vi "Page_Dialog_Read.vi"(6 "ctlReferences":T1, 8 "error in (no error)":errorcluster, 11 "Class in":refnum<class "IB_MSI.lvclass">) -> (0 "error out":errorcluster, 3 "Class out":refnum<class "IB_MSI.lvclass">)   [LabVIEW 2020, in "IB_MSI.lvclass"]
uses:
  <vilib>/AppBuilder/IB_Classes/MSI/IB_MSI.lvclass
  <vilib>/AppBuilder/IB_Classes/MSI/IB_MSI.lvclass/IB_MSI.ctl
  <vilib>/AppBuilder/IB_Classes/Installer/Installer.lvclass
  <resource>/Framework/Providers/Builds/Installer/CDK_sTypeDef_Languages.ctl
  <resource>/Framework/Providers/Builds/Installer/Pages/controls/IB_UI_Page_Dialog_Info_References.ctl
  <resource>/Framework/Providers/Common/provcom_BrowseProjectFile2.ctl
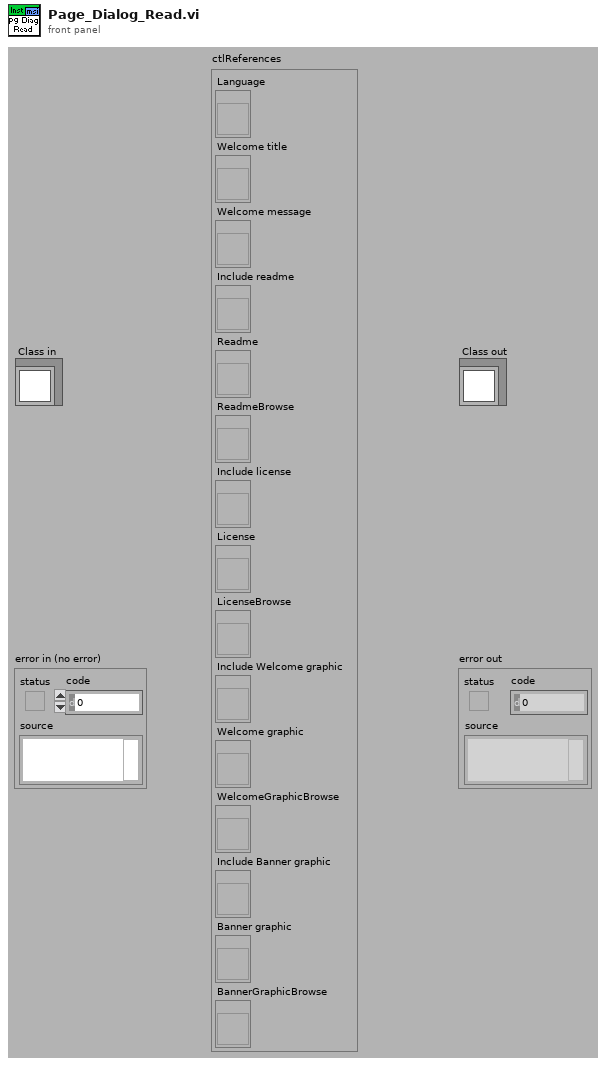
[diagram p1: front panel]
types:
  T1 = typedef "IB_UI_Page_Dialog_Info_References.ctl" = cluster{"Language":refnum<vi>, "Welcome title":refnum<vi>, "Welcome message":refnum<vi>, "Include readme":refnum<vi>, "Readme":refnum<vi>, "ReadmeBrowse":refnum<vi>, "Include license":refnum<vi>, "License":refnum<vi>, "LicenseBrowse":refnum<vi>, "Include Welcome graphic":refnum<vi>, "Welcome graphic":refnum<vi>, "WelcomeGraphicBrowse":refnum<vi>, "Include Banner graphic":refnum<vi>, "Banner graphic":refnum<vi>, "BannerGraphicBrowse":refnum<vi>}
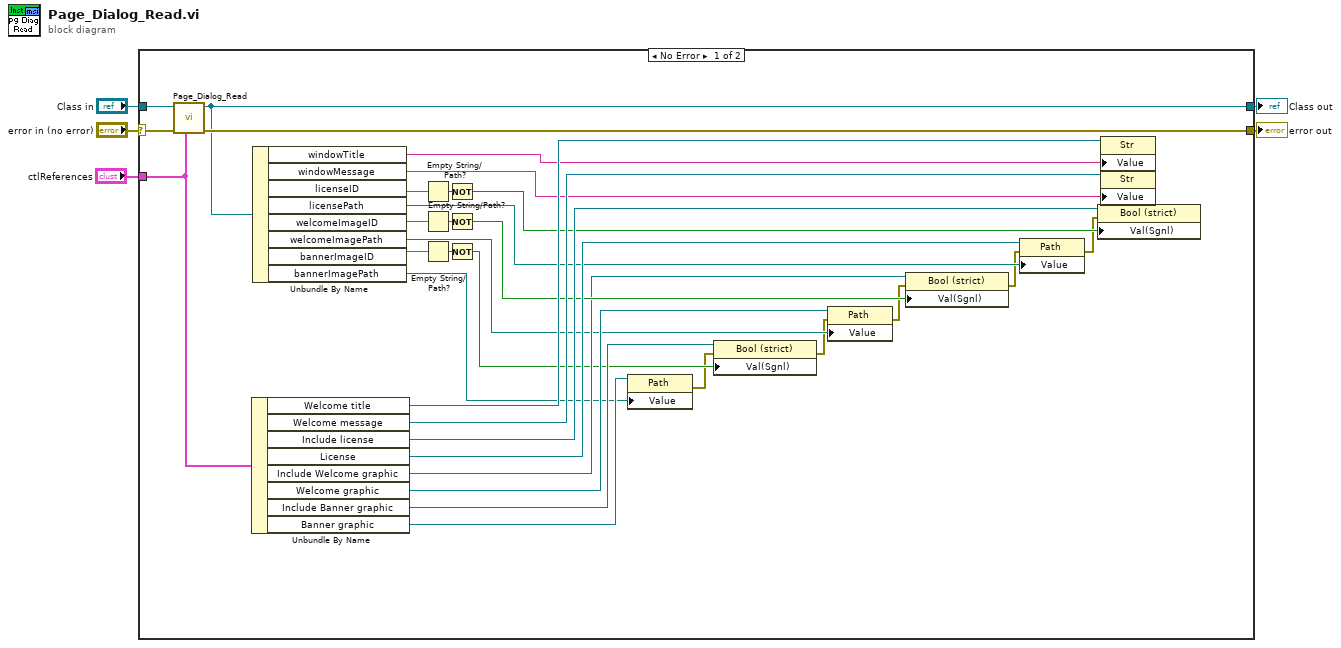
[diagram p0: block diagram]
diagram:
  n1 = case shown="No Error" "error in (no error)" {
    selector: "error in (no error)" -> [w34 w39]
    tunnel: [w33 w39] -> w4
    tunnel: [w11 w38] -> w2
    tunnel: "Class in" -> [w35 w38]
    tunnel: "ctlReferences" -> [w32 _]
    frame No Error {
      n2 = call-parent "Page_Dialog_Read.vi"("ctlReferences"=w32, "error in (no error)"=w34, "Class in"=w35) -> ("error out"=w33:errorcluster, "Class out"=w11:refnum<class "IB_MSI.lvclass">)  [unwired: 7 out]
      n3 = Unbundle By Name(w32) -> ("Welcome title"=w37:refnum<vi>, "Welcome message"=w31:refnum<vi>, "Include license"=w29:refnum<vi>, "License"=w28:refnum<vi>, "Include Welcome graphic"=w18:refnum<vi>, "Welcome graphic"=w17:refnum<vi>, "Include Banner graphic"=w16:refnum<vi>, "Banner graphic"=w15:refnum<vi>)
      n4 = Unbundle By Name(w11) -> ("windowTitle"=w36:string, "windowMessage"=w30:string, "licenseID"=w27:string, "licensePath"=w22:path, "welcomeImageID"=w21:string, "welcomeImagePath"=w14:path, "bannerImageID"=w19:string, "bannerImagePath"=w12:path)
      n5 = Empty String/Path?(string/path=w27) -> (empty?=w26:bool)
      n6 = Empty String/Path?(string/path=w21) -> (empty?=w24:bool)
      n7 = Empty String/Path?(string/path=w19) -> (empty?=w23:bool)
      n8 = Not(x=w26) -> (.not. x?=w25:bool)
      n9 = Not(x=w24) -> (.not. x?=w20:bool)
      n10 = Not(x=w23) -> (.not. x?=w13:bool)
      n11 = property class="Path"(reference=w15, "Value"=w12) -> (error out=w10:errorcluster)  [unwired: 1 in, 1 out]
      n12 = property class="Bool (strict)"(reference=w16, error in=w10, "Val(Sgnl)"=w13) -> (error out=w9:errorcluster)  [unwired: 1 out]
      n13 = property class="Path"(reference=w17, error in=w9, "Value"=w14) -> (error out=w8:errorcluster)  [unwired: 1 out]
      n14 = property class="Bool (strict)"(reference=w18, error in=w8, "Val(Sgnl)"=w20) -> (error out=w7:errorcluster)  [unwired: 1 out]
      n15 = property class="Path"(reference=w28, error in=w7, "Value"=w22) -> (error out=w6:errorcluster)  [unwired: 1 out]
      n16 = property class="Bool (strict)"(reference=w29, error in=w6, "Val(Sgnl)"=w25) -> ()  [unwired: 2 out]
      n17 = property class="Str"(reference=w37, "Value"=w36) -> ()  [unwired: 1 in, 2 out]
      n18 = property class="Str"(reference=w31, "Value"=w30) -> ()  [unwired: 1 in, 2 out]
    }
    frame Error {
    }
  }
  "error out" <- w4
  "Class out" <- w2
